vi "ctx ap set io value.vi"(7 "output_value":u32, 9 "gpio_pin":u32(ring) items=["APDM_AP_GPIO_0", "APDM_AP_ANALOG_OUT_0", "APDM_AP_ANALOG_IN_0"], 10 "ap_id":u32, 11 "context":u32) -> (2 "function return":i32, 3 "context out":u32)   [LabVIEW 2019, in "apdm.lvlib"]
doc: "APDM_EXPORT int apdm_ctx_ap_set_io_value(apdm_ctx_t context, const uint32_t ap_id, const apdm_ap_gpio_pin_t gpio_pin, const uint32_t output_value);"
uses:
  apdm.lvlib
  Lee Lab/CP FES Walking 2018/Code/Working/LabVIEW/apdm.dll
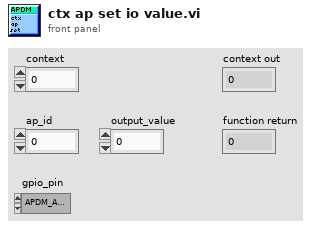
[diagram p1: front panel]
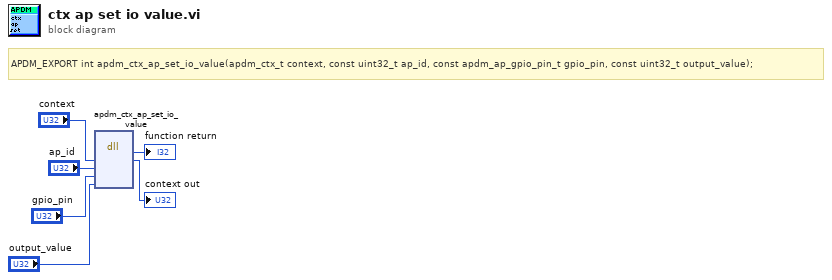
[diagram p0: block diagram]
diagram:
  # "APDM_EXPORT int apdm_ctx_ap_set_io_value(apdm_ctx_t context, const uint32_t ap_id, const apdm_ap_gpio_pin_t gpio_pin, const uint32_t output_value);"
  n1 = dll-call lib="C:/Users/jfalesi/Dropbox/Lee Lab/CP FES Walking 2018/Code/Working/LabVIEW/apdm.*" fn="apdm_ctx_ap_set_io_value"("context"="context", "ap_id"="ap_id", "gpio_pin"="gpio_pin", "output_value"="output_value") -> (→"function return":i32, "context"=→"context out":u32)  [unwired: 6 in, 2 out]
